vi "blaze.vi"(2 "String 2":string, 3 "String":string) -> (0 "String 5":string, 1 "String 4":string)   [LabVIEW 2017]
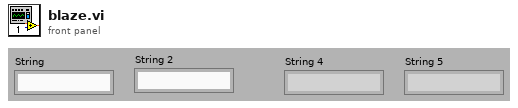
[diagram p1: front panel]
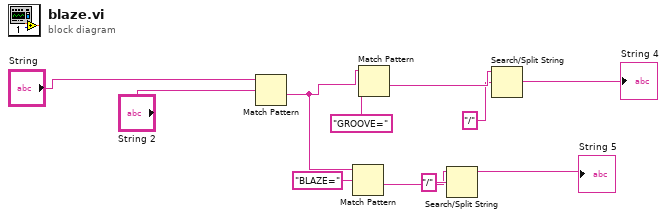
[diagram p0: block diagram]
diagram:
  n1 = Match Pattern(string="String", regular expression="String 2") -> (after substring=w8:string)  [unwired: 1 in, 3 out]
  n2 = Match Pattern(string=w8, regular expression="BLAZE=") -> (after substring=w6:string)  [unwired: 1 in, 3 out]
  n3 = Match Pattern(string=w8, regular expression="GROOVE=" ("search string/char (-)")) -> (after substring=w4:string)  [unwired: 1 in, 3 out]
  n4 = Search/Split String(string=w6, search string/char (-)="/") -> (substring before match=→"String 5":string)  [unwired: 1 in, 2 out]
  n5 = Search/Split String(string=w4, search string/char (-)="/") -> (substring before match=→"String 4":string)  [unwired: 1 in, 2 out]
